vi "RSZVB Set Loss At DC.vi"(7 "Loss At DC (0.0 dB)":dbl format="%^.3e", 8 "error in (no error)":errorcluster {"code" format="%.0x"}, 9 "Port (1)":i32=1, 10 "Channel (1)":i32=1, 11 "VISA session":refnum<visa-resource-name>) -> (0 "error out":errorcluster {"code" format="%.0x"}, 3 "dup VISA session":refnum<visa-resource-name>)   [LabVIEW 2011]
doc: "This VI defines the frequency-independent part (DC value) of the offset loss.\n\nRemote-control command(s):\n[SENSe<Ch>:]CORRection:LOSS<port_no> <DC_loss>"
uses:
  _utility/RSZVB Global Data.vi
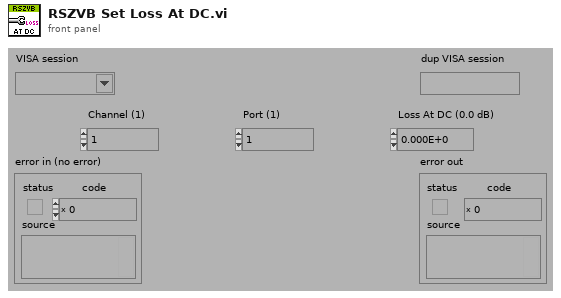
[diagram p1: front panel]
types:
  T1 = cluster{"Error Checking (T: On)":bool, "Installed Options":string[], "Data Valid?":bool, "Ports":i32, "Model":string[], "Option Checking (T: On)":bool}[]
  T2 = cluster{"Error Checking (T: On)":bool, "Installed Options":string[], "Data Valid?":bool, "Ports":i32, "Model":string[], "Option Checking (T: On)":bool}
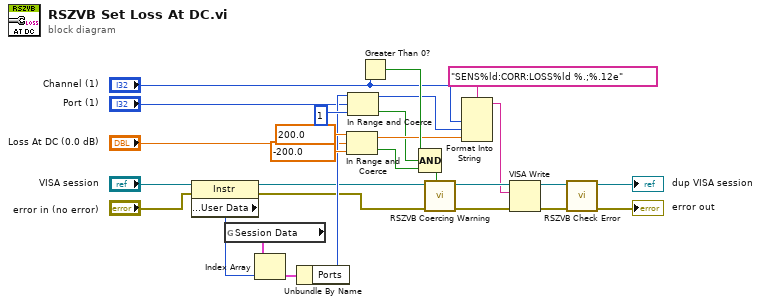
[diagram p0: block diagram]
diagram:
  n1 = property class="Instr"(reference="VISA session", error in="error in (no error)") -> (reference out=w11:refnum<visa-resource-name>, error out=w12:errorcluster, "General Settings:User Data"=w15:u32)
  n2 = global read "RSZVB Global Data.vi" "Session Data"() -> (w16:T1)
  n3 = Index Array(array=w16, index=w15) -> (element=w17:T2)
  n4 = Unbundle By Name(w17) -> ("Ports"=w13:i32)
  n5 = In Range and Coerce(upper limit=200.0, x="Loss At DC (0.0 dB)", lower limit=-200.0) -> (coerced(x)=w18:dbl, In Range?=w9:bool)
  n6 = In Range and Coerce(upper limit=w13, x="Port (1)", lower limit=1) -> (coerced(x)=w10:i32, In Range?=w8:bool)
  n7 = Greater Than 0?(x="Channel (1)") -> (x > 0?=w21:bool)
  n8 = Compound Arithmetic op=AND(w21, w8, w9) -> (w23:bool)
  n9 = call "RSZVB Coercing Warning.vi"("In Range?"=w23, "error in (no error)"=w12, "VISA session"=w11) -> ("error out"=w26:errorcluster, "dup VISA session"=w27:refnum<visa-resource-name>)  [unwired: 7 in]
  n10 = Format Into String(format string="SENS%ld:CORR:LOSS%ld %.;%.12e", "Channel (1)", w10, w18) -> (resulting string=w22:string)  [unwired: 2 in, 1 out]
  n11 = VISA Write(VISA resource name=w27, write buffer=w22, error in (no error)=w26) -> (VISA resource name out=w24:refnum<visa-resource-name>, error out=w25:errorcluster)  [unwired: 1 out]
  n12 = call "RSZVB Check Error.vi"("error in (no error)"=w25, "VISA session"=w24) -> ("error out"=→"error out":errorcluster, "dup VISA session"=→"dup VISA session":refnum<visa-resource-name>)  [unwired: 8 in]
